vi "TEST_SimResistor.vi"() -> ()   [LabVIEW 2024]
doc: "This VI is used to test the Spec LUT (Look Up Table) Select ChA!ChB and Drain!Fill\nShould produce the spec index for the level entered.\nNote: Meausre shows the value whre Measure R is enabled."
uses:
  Control Definitions/Def FullCfg.ctl
  Control Definitions/Def BenchCfg.ctl
  Control Definitions/Def PumpCtlRefs.ctl
  Control Definitions/Def_PumpSpeed.ctl
  Control Definitions/Def Bench Status.ctl
  Control Definitions/Def Spec RNG.ctl
  Control Definitions/Ded LUT_Status.ctl
panel:
  in  "Test Index":i32
  in  "Full Cfg 2":T1={"Bench Config"={"Name"="OLR001", {"Step Levels"=0.05, "Tolerance"=0.01, "Sample Rate"=0.05, "Resistor"=100.0, "M Level Cal"=1.0, "[B Level Cal"=0.0, "Max Fill Rate"=0.002, "Empty Inches"=8.0, "Full Inches"=2.6}}, "Test Value Table "=[[98.0, 102.0, 8.5, 8.5, 8.5, 8.5, 98.0, 102.0, 8.5, 8.5, 8.5, 8.5], [98.0, 102.0, 7.91, 8.01, 7.55, 7.65, 98.0, 102.0, 7.685, 7.785, 7.325, 7.425], [197.0, 203.0, 7.46, 7.56, 7.1, 7.2, 197.0, 203.0, 7.235, 7.335, 6.875, 6.975], [296.0, 304.0, 7.01, 7.11, 6.65, 6.75, 296.0, 304.0, 6.785, 6.885, 6.425, 6.525], [395.0, 405.0, 6.56, 6.66, 6.2, 6.3, 395.0, 405.0, 6.335, 6.435, 5.975, 6.075], [494.0, 506.0, 6.11, 6.21, 5.75, 5.85, 494.0, 506.0, 5.885, 5.985, 5.525, 5.625], [593.0, 607.0, 5.66, 5.76, 5.3, 5.4, 593.0, 607.0, 5.435, 5.535, 5.075, 5.175], [692.0, 708.0, 5.21, 5.31, 4.85, 4.95, 692.0, 708.0, 4.985, 5.085, 4.625, 4.725], [791.0, 809.0, 4.76, 4.86, 4.4, 4.5, 791.0, 809.0, 4.535, 4.635, 4.175, 4.275], [890.0, 910.0, 4.31, 4.41, 3.95, 4.05, 890.0, 910.0, 4.085, 4.185, 3.725, 3.825], [989.0, 1011.0, 3.86, 3.96, 3.5, 3.6, 989.0, 1011.0, 3.635, 3.735, 3.275, 3.375], [1088.0, 1112.0, 3.41, 3.51, 3.05, 3.15, 1088.0, 1112.0, 3.185, 3.285, 2.825, 2.925], [1088.0, 1112.0, 2.5, 2.5, 2.5, 2.5, 1088.0, 1112.0, 2.5, 2.5, 2.5, 2.5]], "Table Col Titles"=[["Aohm Lo", "Aohm Hi", "A Fill Lo", "A Fill Hi", "A Drain Lo", "A Drain Hi", "Bohm Lo", "Bohm Hi", "B Fill Lo", "B Fill Hi", "B Drain Lo", "B Drain Hi"]], "cluster"={"Fill "=refnum, "Drain"=refnum, "Level PV"=refnum, "Pump Speed"=refnum, "Run Test"=refnum, "Sim"=refnum, "Jog"=refnum, "Level SP"=refnum}, "Bench Status"={"Pump Status"=refnum, "Instrumnet\n Status"=refnum}}
  in  "stop":bool
  out "Ch B  Ohms":dbl
  out "Ch A  Ohms":dbl
  in  "Drain!Fill":bool
  in  "Level IN inches":dbl
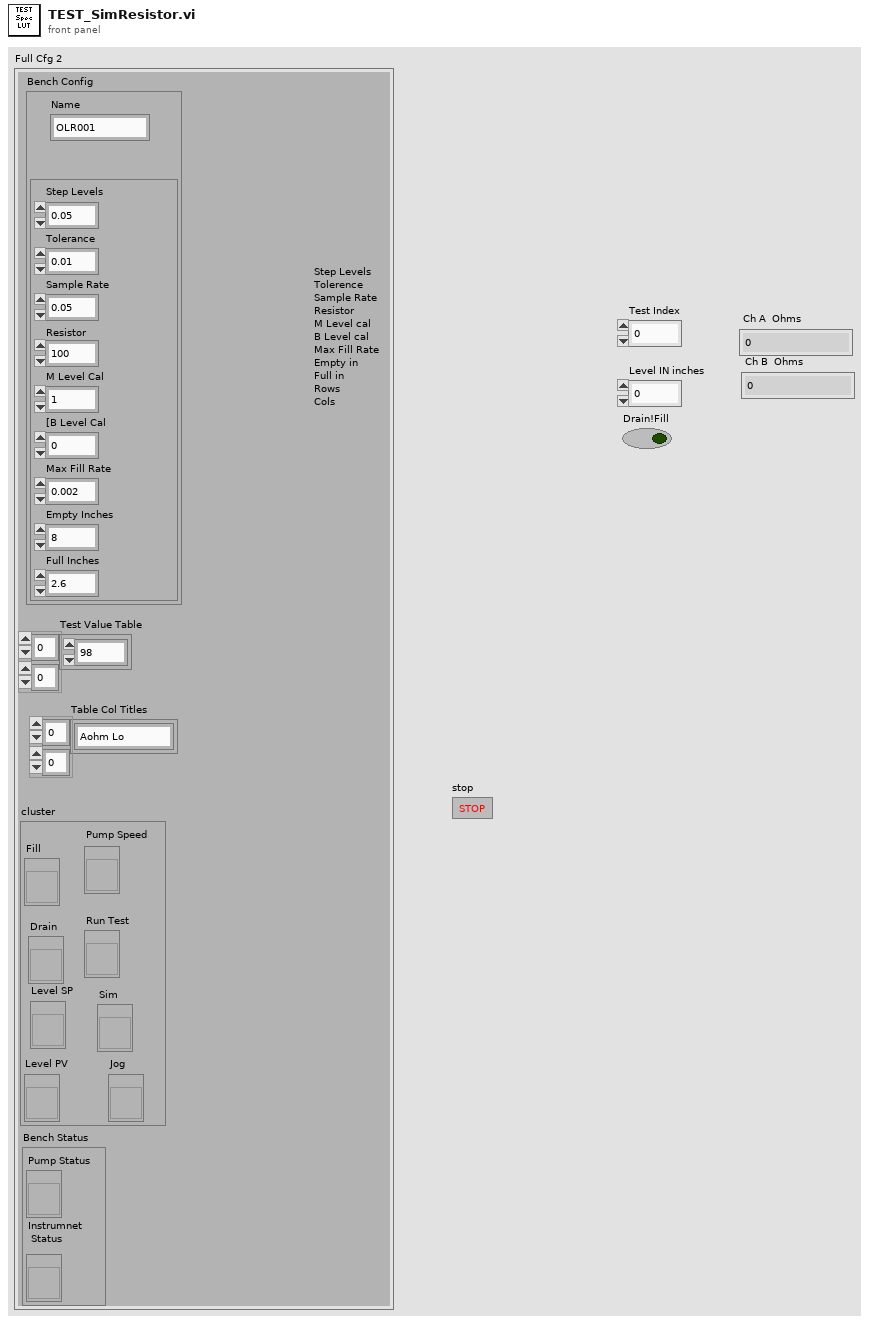
[diagram p1: front panel]
types:
  T1 = typedef "Def FullCfg.ctl" = cluster{"Bench Config":T2, "Test Value Table ":dbl[][], "Table Col Titles":string[][], "cluster":T3, "Bench Status":T4}
  T2 = typedef "Def BenchCfg.ctl" = cluster{"Name":string, cluster{"Step Levels":dbl, "Tolerance":dbl, "Sample Rate":dbl, "Resistor":dbl, "M Level Cal":dbl, "[B Level Cal":dbl, "Max Fill Rate":dbl, "Empty Inches":dbl, "Full Inches":dbl}}
  T3 = typedef "Def PumpCtlRefs.ctl" = cluster{"Fill ":refnum<vi>, "Drain":refnum<vi>, "Level PV":refnum<vi>, "Pump Speed":refnum<vi>, "Run Test":refnum<vi>, "Sim":refnum<vi>, "Jog":refnum<vi>, "Level SP":refnum<vi>}
  T4 = typedef "Def Bench Status.ctl" = cluster{"Pump Status":refnum<vi>, "Instrumnet\n Status":refnum<vi>}
  T5 = typedef "Def Spec RNG.ctl" = cluster{"Specs":dbl[], "LUT Status":T6}
  T6 = typedef "Ded LUT_Status.ctl" = cluster{"ChA/!ChB":bool, "Drain/!Fill":bool, "In Range?":bool, "Switch Range?":bool, "Measure R?":bool, "Vaild R?":bool, "Index(n)":i32, "Index(n-1)":i32, "Index Max":i32}
  T7 = cluster{"Spec RNG Out":T5[], "cluster":T3, "TEST State Out":u16, "Index":i32, "X>Pos":bool}
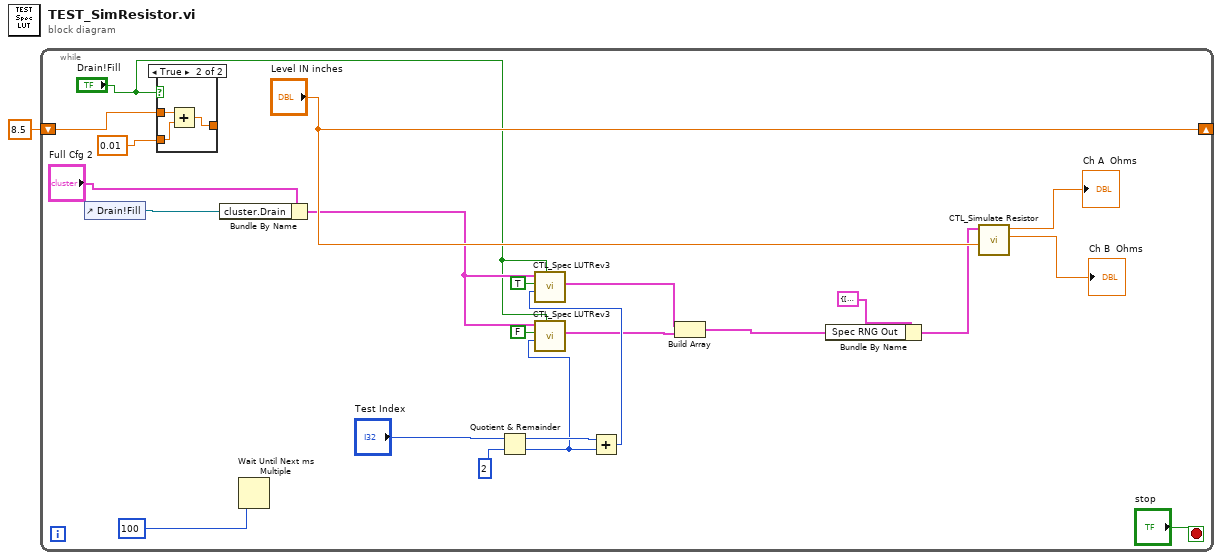
[diagram p0: block diagram]
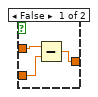
[diagram p2: hidden frame]
diagram:
  n1 = while {
    shift-right: ["Level IN inches"] -> _
    shift-left: 8.5 ("Level IN inches") -> [w19]
    stop <- "stop" stop-if-true
    n2 = control-ref of="Drain!Fill"() -> (w24:refnum<vi>)
    n3 = case shown="True" "Drain!Fill" {
      tunnel: w19 -> [w27 w30]
      tunnel: 0.01 -> [w26 w28]
      tunnel: [w25 w29] -> _
      frame False {
        n4 = Subtract(x=w27, y=w26) -> (x-y=w25:dbl)
      }
      frame True {
        n5 = Add(x=w30, y=w28) -> (x+y=w29:dbl)
      }
    }
    n6 = Bundle By Name(cluster="Full Cfg 2", "cluster.Drain"=w24) -> (w7:T1)
    n7 = Wait Until Next ms Multiple(millisecond multiple=u32 100) -> ()  [unwired: 1 out]
    n8 = Quotient & Remainder(x="Test Index", y=2) -> (x-y*floor(x/y)=w14:i32, floor(x/y)=w8:i32)
    n9 = call "CTL_Spec LUTRev3.vi"("Drain!Fill"="Drain!Fill", "Index"=w8, "ChA/!ChB"=FALSE, "Full Cfg"=w7) -> ("Spec Range Out"=w9:T5)  [unwired: 4 in, 3 out]
    n10 = Add(x=w14, y=w8) -> (x+y=w11:i32)
    n11 = call "CTL_Spec LUTRev3.vi"("Drain!Fill"="Drain!Fill", "Index"=w11, "ChA/!ChB"=TRUE, "Full Cfg"=w7) -> ("Spec Range Out"=w10:T5)  [unwired: 4 in, 3 out]
    n12 = Build Array(w10, w9) -> (w3:T5[])
    n13 = Bundle By Name(cluster=T7 {"Spec RNG Out"=[], "cluster"={"Fill "=refnum, "Drain"=refnum, "Level PV"=refnum, "Pump Speed"=refnum, "Run Test"=refnum, "Sim"=refnum, "Jog"=refnum, "Level SP"=refnum}, "TEST State Out"=0, "Index"=0, "X>Pos"=FALSE}, "Spec RNG Out"=w3) -> (w2:T7)
    n14 = call "CTL_Simulate Resistor.vi"("Level IN"="Level IN inches", "Specs IN"=w2) -> ("Ch B  Ohms"=→"Ch B  Ohms":dbl, "Ch A  Ohms"=→"Ch A  Ohms":dbl)  [unwired: 7 in, 1 out]
  }
